vi "RIGOL DP800 Series Output DC Volts.vi"() -> ()   [LabVIEW 2013]
doc: "This example shows how to configure the instrument's output voltage level, over current protection, and over voltage protection. The actual voltage level and actual current level are returned as well as whether over voltage protection (OVP) or over current protection (OCP) has been tripped."
uses:
  <instrlib>/RIGOL DP800 Series/Public/Channels.ctl
  <instrlib>/RIGOL DP800 Series/RIGOL DP800 Series.lvlib
panel:
  out "Current":dbl(graph)
  out "Voltage":dbl(graph)
  in  "Channel (0: 30V Channel)":T1 caption="Channel (0: +6V)" items=["30V/3A Channel", "30V/3A Channel", "5V/3A Channel"]
  out "Actual Power Level (W)":dbl caption="Actual Power Level" format="%#.6f"
  in  "Enable OVP (T: Enable)":bool=TRUE
  in  "Stop Output":bool
  in  "Behavior (0: Regulate)":u16(ring) items=["Regulate", "Trip"]
  in  "Voltage Limit (0V)":dbl format="%.2f"
  out "Actual Current Sourced (A)":dbl caption="Actual Current Limit (A)" format="%#.6f"
  out "Actual Voltage Level (V)":dbl format="%#.6f"
  in  "Voltage Level (0.0 V)":dbl format="%.2f"
  in  "Current Limit (0A)":dbl format="%.2f"
  in  "VISA resource name":refnum<visa-resource-name>
  # "Modified from the DP1308A VIs from http://sine.ni.com/apps/utf8/niid_web_display.model_page?p_model_id=19034"
  # "Over Voltage Protection"
  # "Over Current Protection"
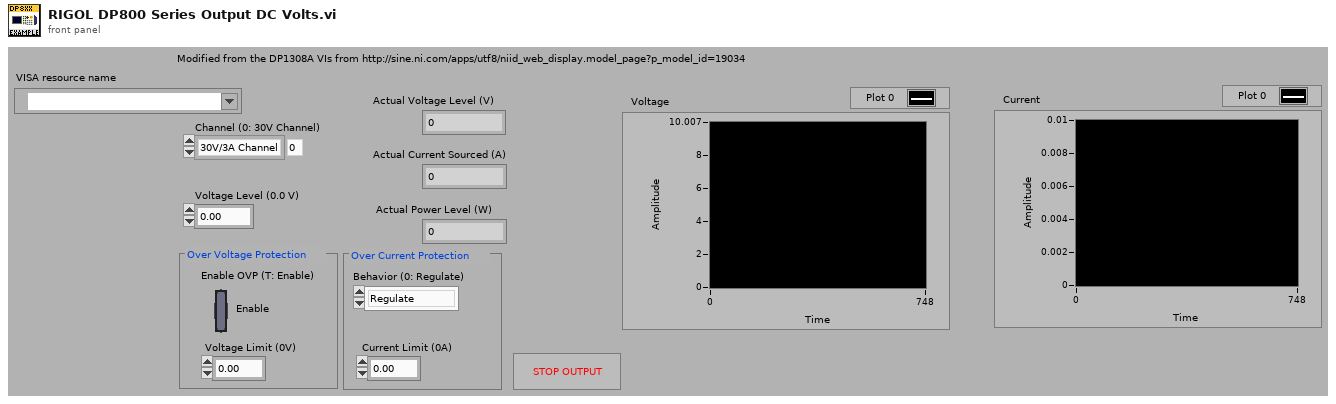
[diagram p1: front panel]
types:
  T1 = typedef "RIGOL DP800 Series.lvlib/Channels.ctl" = i32
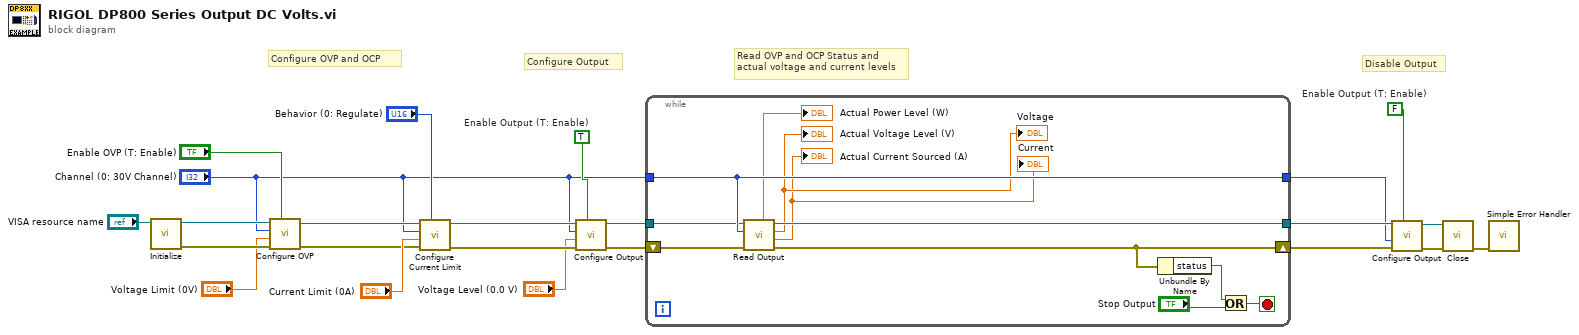
[diagram p0: block diagram]
diagram:
  w11 = FALSE  # Enable Output (T: Enable)
  w12 = TRUE  # Enable Output (T: Enable)
  # "Disable Output"
  # "Read OVP and OCP Status and\nactual voltage and current levels"
  # "Configure Output"
  # "Configure OVP and OCP"
  n1 = call <instrlib>:"Initialize.vi"("VISA resource name"="VISA resource name") -> ("error out"=w8:errorcluster, "VISA resource name out"=w9:refnum<visa-resource-name>)  [unwired: 9 in]
  n2 = call <instrlib>:"Configure OVP.vi"("Enable OVP (T: Enable)"="Enable OVP (T: Enable)", "error in (no error)"=w8, "Voltage Limit (6.5 V)"="Voltage Limit (0V)", "Channel (0: 30V Channel)"="Channel (0: 30V Channel)", "VISA resource name"=w9) -> ("error out"=w7:errorcluster, "VISA resource name out"=w6:refnum<visa-resource-name>)  [unwired: 5 in]
  n3 = call <instrlib>:"Configure Current Limit.vi"("Behavior (0: Regulate)"="Behavior (0: Regulate)", "error in (no error)"=w7, "Current Limit (5.0 A)"="Current Limit (0A)", "Channel (0: 30V Channel)"="Channel (0: 30V Channel)", "VISA resource name"=w6) -> ("error out"=w21:errorcluster, "VISA resource name out"=w22:refnum<visa-resource-name>)  [unwired: 5 in]
  n4 = call <instrlib>:"Configure Output.vi"("Enable Output (T: Enable)"=w12, "error in (no error)"=w21, "Voltage Level (0.0 V)"="Voltage Level (0.0 V)", "Channel (0: 30V Channel)"="Channel (0: 30V Channel)", "VISA resource name"=w22) -> ("error out"=w18:errorcluster, "VISA resource name out"=w19:refnum<visa-resource-name>)  [unwired: 5 in]
  n5 = while {
    tunnel: w19 -> [w28]
    tunnel: [w34] -> w17
    tunnel: "Channel (0: 30V Channel)" -> [w33]
    tunnel: [w33] -> w3
    shift-right: [w30] -> w16
    shift-left: w18 -> [w27]
    stop <- w32 stop-if-true
    n6 = call <instrlib>:"Read Output.vi"("error in (no error)"=w27, "Channel (0: 30V Channel)"=w33, "VISA resource name"=w28) -> ("error out"=w30:errorcluster, "Actual Current Level (A)"=→"Actual Current Sourced (A)" →"Current":dbl, "Actual Voltage Level (V)"=→"Actual Voltage Level (V)" →"Voltage":dbl, "VISA resource name out"=w34:refnum<visa-resource-name>, "Actual Power Level (W)"=→"Actual Power Level (W)":dbl)  [unwired: 4 in]
    n7 = Unbundle By Name(w30) -> ("status"=w29:bool)
    n8 = Or(x=w29, y="Stop Output") -> (x .or. y?=w32:bool)
  }
  n9 = call <instrlib>:"Configure Output.vi"("Enable Output (T: Enable)"=w11, "error in (no error)"=w16, "Voltage Level (0.0 V)"=w3, "VISA resource name"=w17) -> ("error out"=w14:errorcluster, "VISA resource name out"=w15:refnum<visa-resource-name>)  [unwired: 6 in]
  n10 = call <instrlib>:"Close.vi"("error in (no error)"=w14, "VISA resource name"=w15) -> ("error out"=w10:errorcluster)  [unwired: 9 in]
  n11 = call <vilib>:"Simple Error Handler.vi"("error in (no error)"=w10) -> ()  [unwired: 1 in, 8 out]
